vi "Hardware-DCM-23XX-Cmd.vi"(8 "error in (no error)":errorcluster, 9 "LoopCount":i32, 10 "LoopPeriod [usec]":u32, 11 "DSI Reference":refnum<class "DCM-DSI.lvclass">) -> (0 "error out":errorcluster, 3 "DSI Reference":refnum<class "DCM-DSI.lvclass">)   [LabVIEW 2016, in "DSI-RT.lvlib"]
uses:
  DSI-RT.lvlib
  Classes/DCM-DSI/DCM-DSI.lvclass
  Classes/DCM-DSI/Read DCM Ref.vi
  Classes/DCM-DSI/Write dt.vi
  Classes/DCM-DSI/Write LoopCount.vi
  <vilib>/Powertrain Controls/Device Drivers/DCM/Rev0/RT/Read System ADC.vi
  Classes/DCM-DSI/Write EPTx Data.vi
  Classes/DCM-DSI/Write Knock Results.vi
  Classes/DCM-DSI/Write System ADC.vi
  <vilib>/Powertrain Controls/Device Drivers/DCM/Rev0/RT/DCM - RT.lvclass
  <vilib>/addons/Software Calibration Management/xSCM/CalPoint.xnode
  <vilib>/addons/Software Calibration Management/xSCM/FaultPoint.xnode
  <vilib>/addons/Software Calibration Management/xSCM/ni_scm.dll
  <vilib>/Powertrain Controls/Device Drivers/DCM/Tools/RT/DCM - RT - Tools.lvlib
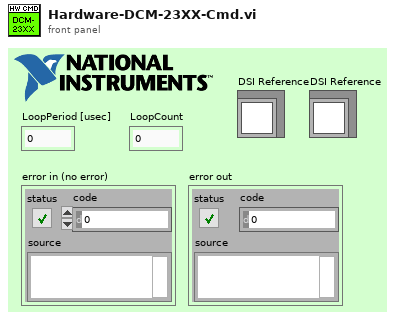
[diagram p1: front panel]
types:
  T1 = typedef "DCM - RT.lvclass/System ADC.ctl" = cluster{"AI 1 [V]":sgl, "AI 2 [V]":sgl, "AI 3 [V]":sgl, "AI 4 [V]":sgl, "AI 5 [V]":sgl, "AI 6 [V]":sgl, "AI 7 [V]":sgl, "AI 8 [V]":sgl, "AI 9 [V]":sgl, "AI 10 [V]":sgl, "AI 11 [V]":sgl, "AI 12 [V]":sgl, "Temp HH 1-6 [C]":sgl, "Temp HH 7-12 [C]":sgl, "Temp DI A [C]":sgl, "Temp DI Zener A [C]":sgl, "Temp DI B [C]":sgl, "Temp DI Zener B [C]":sgl, "Temp CPU [C]":sgl, "Temp Fan Intake [C]":sgl, "Temp Secondary A [C]":sgl, "Temp Primary A [C]":sgl, "Temp Boost B [C]":sgl, "Primary Range [V]":sgl, "Primary A1A2 [V]":sgl, "Primary A3A4 [V]":sgl, "Primary B3B4 [V]":sgl, "Primary B1B2 [V]":sgl, "Secondary A1A2 [V]":sgl, "Secondary A3A4 [V]":sgl, "Secondary B3B4 [V]":sgl, "Secondary B1B2 [V]":sgl, "Ext HV A [V]":sgl, "Ext HV B [V]":sgl, "FET Driver [V]":sgl, "Fan [V]":sgl, "Battery [V]":sgl, "DRVP [V]":sgl, "Key [V]":sgl, "DI Zener A [V]":sgl, "DI Zener B [V]":sgl, "Pump Zener A [V]":sgl, "Pump Zener B [V]":sgl, "MPRD [V]":sgl}
  T2 = typedef "EPTx - RevA - RT.lvlib/EPTxData.ctl" = cluster{"Sync":bool, "CurrentCAD":sgl, "Speed [RPM]":sgl, "Config":bool, "Rcvg Primary":bool, "Stall":bool, "Overflow":bool, "Ratio Error":bool, "Pattern Error":bool, "Aux Warning":bool, "Watchdog Error":bool}
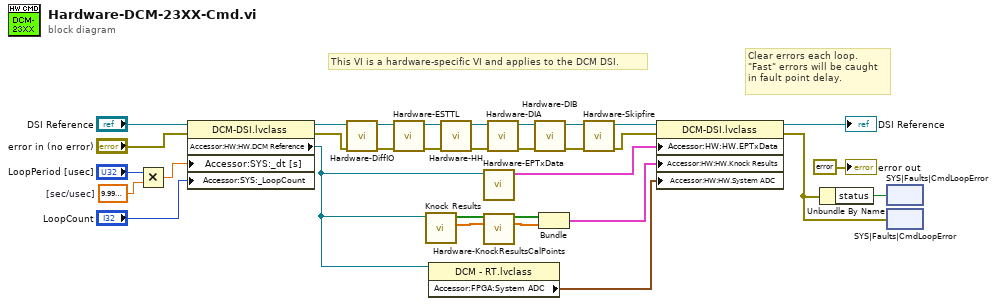
[diagram p0: block diagram]
diagram:
  w29 = sgl 1e-06  # [sec/usec]
  # "Clear errors each loop.\n\"Fast\" errors will be caught\nin fault point delay."
  # "This VI is a hardware-specific VI and applies to the DCM DSI."
  n1 = Multiply(x="LoopPeriod [usec]", y=w29) -> (x*y=w24:sgl)
  n2 = property class="DCM-DSI.lvclass"(reference="DSI Reference", error in="error in (no error)", "Accessor:SYS:_dt [s]"=w24, "Accessor:SYS:_LoopCount"="LoopCount") -> (reference out=w11:refnum<class "DCM-DSI.lvclass">, error out=w8:errorcluster, "Accessor:HW:HW.DCM Reference"=w4:refnum<class "DCM - RT.lvclass">)
  n3 = call "Hardware-DiffIO.vi"("error in (no error)"=w8, "DCM-DSI in"=w11) -> ("error out"=w15:errorcluster, "DCM-DSI out"=w19:refnum<class "DCM-DSI.lvclass">)  [unwired: 8 in]
  n4 = call "Hardware-ESTTL.vi"("error in (no error)"=w15, "DCM-DSI in"=w19) -> ("error out"=w14:errorcluster, "DCM-DSI out"=w18:refnum<class "DCM-DSI.lvclass">)  [unwired: 8 in]
  n5 = call <vilib>:"Knock Results.vi"("DCM Reference"=w4) -> ("Knock Intensity"=w6:sgl[], "Knock"=w7:bool[])  [unwired: 9 in]
  n6 = property class="DCM - RT.lvclass"(reference=w4) -> ("Accessor:FPGA:System ADC"=w20:T1)  [unwired: 1 in, 2 out]
  n7 = call "Hardware-HH.vi"("error in (no error)"=w14, "DCM-DSI in"=w18) -> ("error out"=w13:errorcluster, "DCM-DSI out"=w17:refnum<class "DCM-DSI.lvclass">)  [unwired: 8 in]
  n8 = call "Hardware-EPTxData.vi"("DCM Ref"=w4) -> ("EPTxData"=w26:T2)  [unwired: 10 in]
  n9 = call "Hardware-KnockResultsCalPoints.vi"("Knock"=w7, "Knock Intensity"=w6) -> ()  [unwired: 14 in]
  n10 = call "Hardware-DIA.vi"("error in (no error)"=w13, "DCM-DSI in"=w17) -> ("error out"=w12:errorcluster, "DCM-DSI out"=w16:refnum<class "DCM-DSI.lvclass">)  [unwired: 8 in]
  n11 = call "Hardware-DIB.vi"("error in (no error)"=w12, "DCM-DSI in"=w16) -> ("error out"=w2:errorcluster, "DCM-DSI out"=w3:refnum<class "DCM-DSI.lvclass">)  [unwired: 8 in]
  n12 = Bundle("Knock"=w7, "Knock Intensity"=w6) -> (w5:cluster{"Knock":bool[], "Knock Intensity":sgl[]})  [unwired: 1 in]
  n13 = call "Hardware-Skipfire.vi"("error in (no error)"=w2, "DCM-DSI in"=w3) -> ("error out"=w9:errorcluster, "DCM-DSI out"=w10:refnum<class "DCM-DSI.lvclass">)  [unwired: 8 in]
  n14 = property class="DCM-DSI.lvclass"(reference=w10, error in=w9, "Accessor:HW:HW.EPTxData"=w26, "Accessor:HW:HW.Knock Results"=w5, "Accessor:HW:HW.System ADC"=w20) -> (reference out=→"DSI Reference":refnum<class "DCM-DSI.lvclass">, error out=w1:errorcluster)
  n15 = Unbundle By Name(w1) -> ("status"=w22:bool)
  n16 = xnode "SYS|Faults|CmdLoopError"("Fault"=w22) -> ()
  n17 = xnode "SYS|Faults|CmdLoopError"("Value"=w1) -> ()
  "error out" <- errorcluster {"status"=FALSE, "code"=0, "source"=""} ("error out")
